vi "Write status reference.vi"(8 "error in (no error)":errorcluster, 10 "Status":T1, 11 "SP in":refnum<class "Save messages PGserver.lvclass">) -> (0 "error out":errorcluster, 3 "SP out":refnum<class "Save messages PGserver.lvclass">)   [LabVIEW 2019, in "Save messages PGserver.lvclass"]
uses:
  Save messages PGserver.lvclass
  Modbus/Eth Status/Ctl/Status.ctl
  Modbus/MB_TCP2/MB_TCP_State.ctl
  Save messages PGserver.lvclass/Save messages PGserver.ctl
  Modbus/MB_TCP2/MB_TCP.lvclass
  Modbus/Eth Status/Eth Status.lvlib
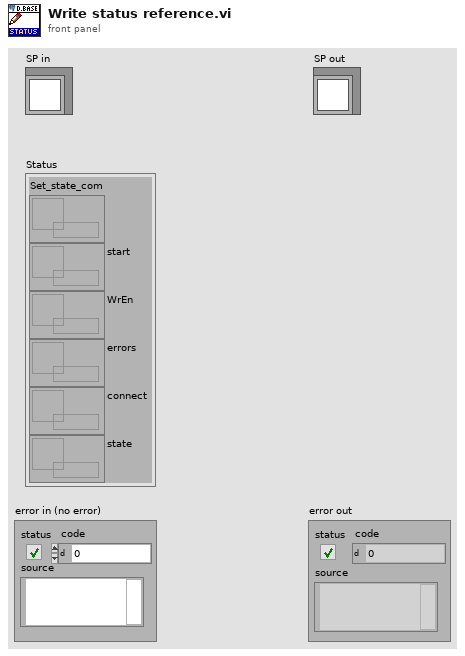
[diagram p1: front panel]
types:
  T1 = typedef "Eth Status.lvlib/Status.ctl" = cluster{"Set_state_com":refnum<data-value>, "start":refnum<data-value>, "WrEn":refnum<data-value>, "errors":refnum<data-value>, "connect":refnum<data-value>, "state":refnum<data-value>}
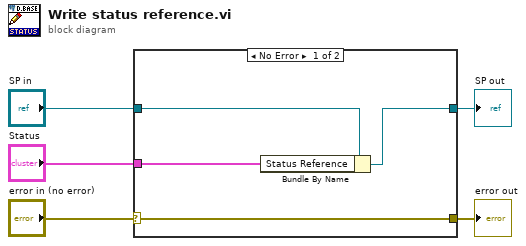
[diagram p0: block diagram]
diagram:
  n1 = case shown="No Error" "error in (no error)" {
    selector: "error in (no error)" -> [w9 w11]
    tunnel: [w9 w11] -> w4
    tunnel: [w8 w10] -> w2
    tunnel: "SP in" -> [w7 w10]
    tunnel: "Status" -> [w6 _]
    frame No Error {
      n2 = Bundle By Name(cluster=w7, "Status Reference"=w6) -> (w8:refnum<class "Save messages PGserver.lvclass">)
    }
    frame Error {
    }
  }
  "error out" <- w4
  "SP out" <- w2
